vi "SRANDMEMBER.vi"(0 "refnum in":refnum<vi>, 1 "Key":string, 5 "Use Count ?":bool, 7 "Count":string, 11 "error in":errorcluster) -> (4 "refnum out":refnum<vi>, 6 "Data":T1, 15 "error out":errorcluster)   [LabVIEW 2023]
uses:
  SubVIs/Controls/redis-data.ctl
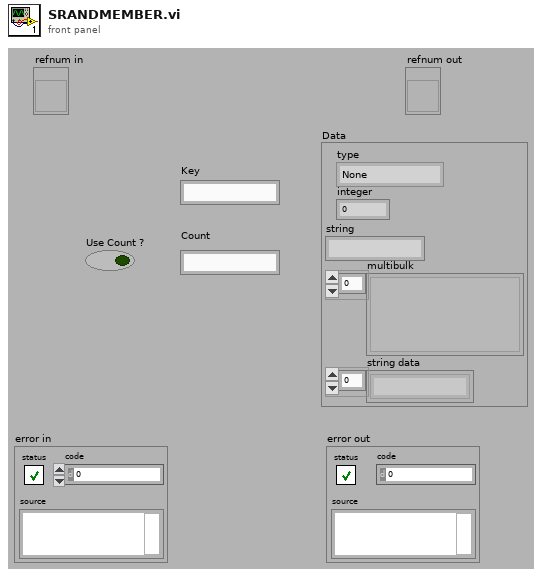
[diagram p1: front panel]
types:
  T1 = typedef "redis-data.ctl" = cluster{"type":enum16{"None", "Error", "Status", "Nil", "Integer", "String", "Multibulk"}, "integer":i64, "string":string, "multibulk":variant[], "string data":string[]}
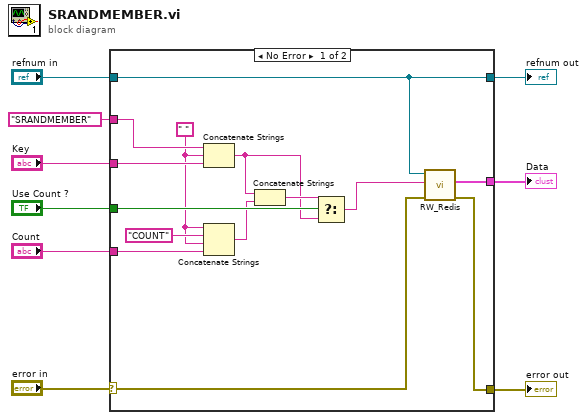
[diagram p0: block diagram]
diagram:
  n1 = case shown="No Error" "error in" {
    selector: "error in" -> [w22 w25]
    tunnel: "Key" -> [w19 _]
    tunnel: "SRANDMEMBER" -> [w23 _]
    tunnel: "refnum in" -> [w11 w24]
    tunnel: [w21 w25] -> w7
    tunnel: [w20 _] -> w1
    tunnel: "Count" -> [w18 _]
    tunnel: "Use Count ?" -> [w16 _]
    tunnel: [w11 w24] -> w3
    frame No Error {
      w15 = " "
      n2 = Concatenate Strings(w23, w15, w19) -> (w13:string)
      n3 = Concatenate Strings(w15, "COUNT", w15, w18) -> (w12:string)
      n4 = Concatenate Strings(w13, w12) -> (w14:string)
      n5 = Select(t=w14, s=w16, f=w13) -> (s? t:f=w10:string)
      n6 = call "RW_Redis.vi"("error in"=w22, "command"=w10, "refnum"=w11) -> ("error out"=w21:errorcluster, "Data"=w20:T1)  [unwired: 7 in]
    }
    frame Error {
    }
  }
  "error out" <- w7
  "Data" <- w1
  "refnum out" <- w3
